vi "Create and Configure Signal Configuration.vi"(8 "error in":errorcluster, 11 "Measurement configuration":T1={"Full scale range"=3.16, "Maximum harmonic"=5, "Analog source resource name"="", "Frequency start"=100.0, "Frequency stop"=20000.0, "Frequency steps"=50, "Frequency spacing"=1, "Amplitude"=1.0, "DC Offset"=0.0, "Measurement duration"=0.001, "Measurement cycles"=10, "Settling time"=0.0, "Settling cycles"=0, "Protocol capture resource name"="", "Data line"=0, "Channel"=0, "Trigger source"=0, "Clock rate"=12288000} {"Settling cycles" min=0 max=5 step=1 format="%.3f"}) -> (0 "error out":errorcluster, 1 "duration":dbl, 3 "signal configuration":refnum<class "SV Discrete Sweep.lvclass">)   [LabVIEW 2021, in "audio_frequencyResponseMeasurement.lvlib"]
uses:
  audio_frequencyResponseMeasurement.lvlib
  Measurement Configuration.ctl
  <vilib>/addons/_NISVFA/_Generation/Signal Generation/SV Discrete Sweep/SV Discrete Sweep.lvclass
  C:/Program Files/National Instruments/LabVIEW 2021/vi.lib/addons/_NISVFA/_Generation/Signal Generation/SV Signal/SV Signal.lvclass
  C:/Program Files/National Instruments/LabVIEW 2021/vi.lib/addons/_NISVFA/_Generation/Signal Generation/SV Function/SV Function.lvclass
  <vilib>/addons/_NISVFA/_Generation/Signal Generation/SV Signal/SV Signal.lvclass/SV Signal.ctl
  <vilib>/addons/_NISVFA/_Generation/Signal Generation/SV Signal/Write Leading Synchronization Pulse Enable.vi
  <vilib>/addons/_NISVFA/_Generation/Signal Generation/SV Signal/Read Total Samples.vi
  <vilib>/addons/_NISVFA/_Generation/Signal Generation/SV Signal/Calculate Number of Remaining Samples.vi
  <vilib>/addons/_NISVFA/_Generation/Signal Generation/SV Discrete Sweep/Configure Frequency Sweep at Constant Amplitude.vi
  <vilib>/addons/_NISVFA/_Generation/Signal Generation/SV Signal/Write Ramp Parameters.vi
  <vilib>/addons/_NISVFA/_Generation/Signal Generation/SV Signal/Write DC Offset.vi
  <vilib>/addons/_NISVFA/_Generation/Signal Generation/SV Signal/Write Measurement Duration.vi
  <vilib>/addons/_NISVFA/_Generation/Signal Generation/SV Function/Write Measurement Cycles.vi
  <vilib>/addons/_NISVFA/_Generation/Signal Generation/SV Signal/Write Pre-Measurement Settling Duration.vi
  <vilib>/addons/_NISVFA/_Generation/Signal Generation/SV Function/Write Pre-Measurement Settling Cycles.vi
  <vilib>/addons/_NISVFA/_Generation/Signal Generation/SV Signal/Read Generation State.vi
  <vilib>/addons/_NISVFA/_Generation/Signal Generation/SV Signal/Read System Timing Model.vi
  <vilib>/addons/_NISVFA/_Generation/Signal Generation/SV Signal/Read Sample Rate.vi
  <vilib>/addons/_NISVFA/_Generation/Signal Generation/SV Signal/SV Signal.lvclass
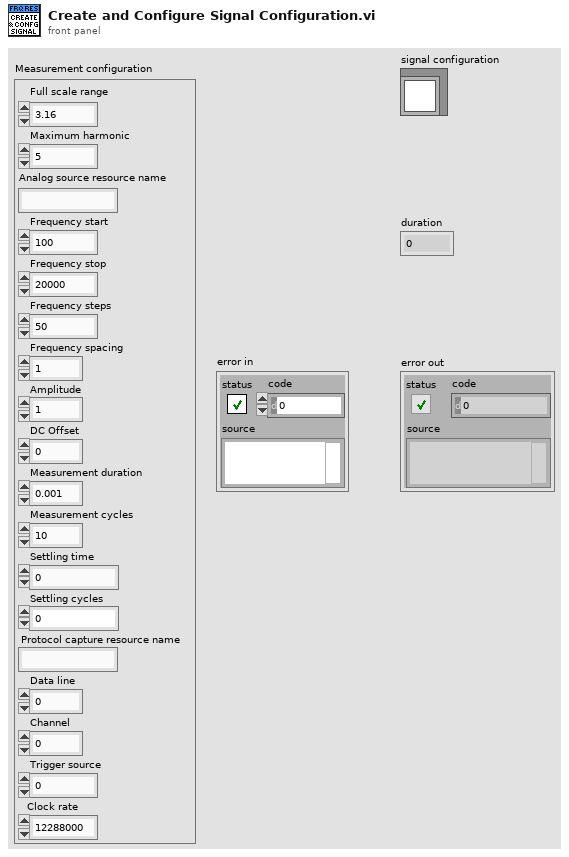
[diagram p1: front panel]
types:
  T1 = typedef "audio_frequencyResponseMeasurement.lvlib/Measurement Configuration.ctl" = cluster{"Full scale range":dbl, "Maximum harmonic":i32, "Analog source resource name":string, "Frequency start":dbl, "Frequency stop":dbl, "Frequency steps":i32, "Frequency spacing":u16, "Amplitude":dbl, "DC Offset":dbl, "Measurement duration":dbl, "Measurement cycles":i32, "Settling time":dbl, "Settling cycles":i32, "Protocol capture resource name":string, "Data line":u16, "Channel":u32, "Trigger source":u16, "Clock rate":u32}
  T2 = cluster{"profile":enum16{"Linear", "Half cosine"}, "durations [s]":cluster{"ramp-up":dbl, "transition":dbl, "ramp-down":dbl}}
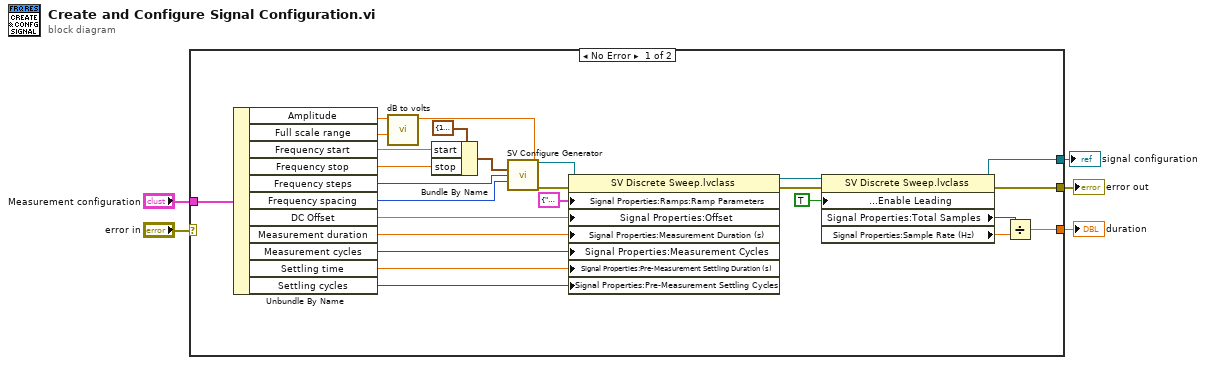
[diagram p0: block diagram]
diagram:
  n1 = case shown="No Error" "error in" {
    selector: "error in" -> [_ w32]
    tunnel: "Measurement configuration" -> [w31 _]
    tunnel: [w8 w32] -> w3
    tunnel: [w7 _] -> w1
    tunnel: [w6 _] -> w2
    frame No Error {
      n2 = Unbundle By Name(w31) -> ("Amplitude"=w29:dbl, "Full scale range"=w30:dbl, "Frequency start"=w26:dbl, "Frequency stop"=w25:dbl, "Frequency steps"=w23:i32, "Frequency spacing"=w22:u16, "DC Offset"=w18:dbl, "Measurement duration"=w17:dbl, "Measurement cycles"=w16:i32, "Settling time"=w15:dbl, "Settling cycles"=w14:i32)
      n3 = call "dB to volts.vi"("Full scale range"=w30, "Voltage(dB)"=w29) -> ("Voltage(volts)"=w28:dbl)  [unwired: 9 in]
      n4 = Bundle By Name(cluster=cluster{"start":dbl, "stop":dbl} {"start"=10.0, "stop"=10000.0} ("frequency range [Hz]"), "start"=w26, "stop"=w25) -> (w24:cluster{"start":dbl, "stop":dbl})
      n5 = call-poly <vilib>:"SV Configure Generator.vi"("amplitude"=w28, "frequency range [Hz]"=w24, "number of steps"=w23, "profile"=w22) -> ("signal configuration"=w19:refnum<class "SV Discrete Sweep.lvclass">, "error out"=w20:errorcluster)  [unwired: 10 in]
      n6 = property class="SV Discrete Sweep.lvclass"(reference=w19, error in=w20, "Signal Properties:Ramps:Ramp Parameters"=T2 {"profile"=enum."Half cosine", "durations [s]"={"ramp-up"=0.01, "transition"=0.0, "ramp-down"=0.01}} ("Ramp Parameters"), "Signal Properties:Offset"=w18, "Signal Properties:Measurement Duration (s)"=w17, "Signal Properties:Measurement Cycles"=w16, "Signal Properties:Pre-Measurement Settling Duration (s)"=w15, "Signal Properties:Pre-Measurement Settling Cycles"=w14) -> (reference out=w12:refnum<class "SV Discrete Sweep.lvclass">, error out=w11:errorcluster)
      n7 = property on="Property Node" class="SV Discrete Sweep.lvclass"(reference=w12, error in=w11, "Signal Properties:Synchronization Pulses:Enable Leading"=TRUE ("Synchronization Pulses:Enable Leading")) -> (reference out=w7:refnum<class "SV Discrete Sweep.lvclass">, error out=w8:errorcluster, "Signal Properties:Total Samples"=w10:i32, "Signal Properties:Sample Rate (Hz)"=w9:dbl)
      n8 = Divide(x=w10, y=w9) -> (x/y=w6:dbl)
    }
    frame Error {
    }
  }
  "error out" <- w3
  "duration" <- w2
  "signal configuration" <- w1
